vi "Obtain number of frames across split AVI2 files.vi"(8 "error in (no error)":errorcluster, 11 "Experiment folder path":path) -> (0 "error out":errorcluster, 3 "Number of Frames (across all split videos of a single channel)":u32)   [LabVIEW 2017]
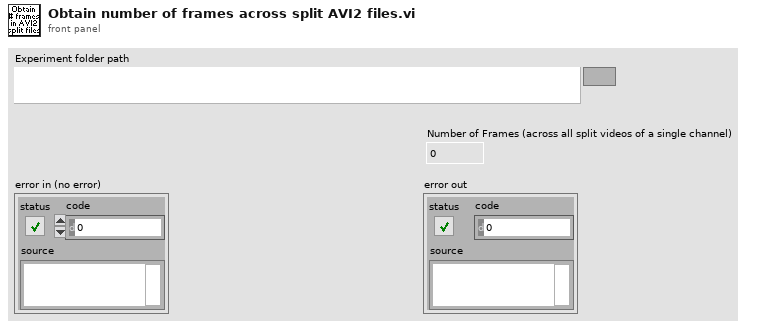
[diagram p1: front panel]
types:
  T1 = typedef "IMAQ AVI2 Refnum.ctl" = refnum<k20>
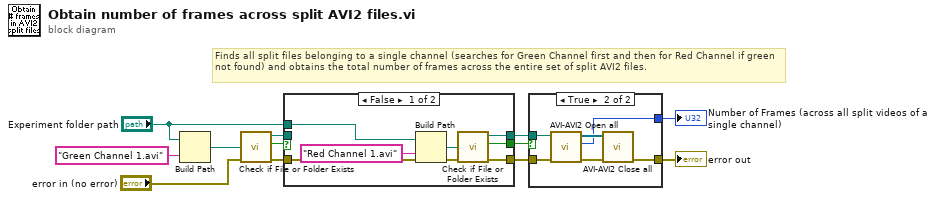
[diagram p0: block diagram]
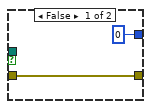
[diagram p2: hidden frame]
diagram:
  # "Finds all split files belonging to a single channel (searches for Green Channel first and then for Red Channel if green not found) and obtains the total number of frames across the entire set of split AVI2 files."
  n1 = Build Path(base path="Experiment folder path", name or relative path="Green Channel 1.avi") -> (appended path=w2:path)
  n2 = call <vilib>:"Check if File or Folder Exists.vi"("error in (no error)"="error in (no error)", "path"=w2) -> ("error out"=w8:errorcluster, "file or folder exists?"=w3:bool, "dup path"=w4:path)  [unwired: 7 in]
  n3 = case shown="False" w3 {
    selector: w3 -> [_ w21]
    tunnel: "Experiment folder path" -> [w19 _]
    tunnel: [w16 w22] -> w6
    tunnel: w4 -> [_ w22]
    tunnel: [w15 w21] -> w5
    tunnel: [w14 w20] -> w7
    tunnel: w8 -> [w13 w20]
    frame False {
      n4 = Build Path(base path=w19, name or relative path="Red Channel 1.avi") -> (appended path=w17:path)
      n5 = call <vilib>:"Check if File or Folder Exists.vi"("error in (no error)"=w13, "path"=w17) -> ("error out"=w14:errorcluster, "file or folder exists?"=w15:bool, "dup path"=w16:path)  [unwired: 7 in]
    }
    frame True {
    }
  }
  n6 = case shown="True" w5 {
    tunnel: w6 -> [_ w30]
    tunnel: w7 -> [w23 w27]
    tunnel: [u32 0 ("Number of Frames (across all split videos)") w26] -> w9
    tunnel: [w23 w25] -> w11
    frame False {
    }
    frame True {
      n7 = call "AVI-AVI2 Open all.vi"("error in (no error)"=w27, "First AVI2 video's Path"=w30) -> ("error out"=w28:errorcluster, "Number of Frames (across all split videos)"=w26:u32, "AVI2 split file refs"=w29:T1[])  [unwired: 5 in, 2 out]
      n8 = call "AVI-AVI2 Close all.vi"("error in (no error)"=w28, "AVI2 ref"=w29) -> ("error out"=w25:errorcluster)  [unwired: 9 in]
    }
  }
  "error out" <- w11
  "Number of Frames (across all split videos of a single channel)" <- w9
